vi "Instr_InitObject.vi"(8 "error in (no error)":errorcluster, 9 "Instrument Configuration":variant, 10 "Instrument address":refnum<visa-resource-name>, 11 "LXIPXISwitching in":refnum<class "LXIPXISwitching.lvclass">) -> (0 "error out":errorcluster, 3 "LXIPXISwitching out":refnum<class "LXIPXISwitching.lvclass">)   [LabVIEW 2019, in "LXIPXISwitching.lvclass"]
uses:
  LXIPXISwitching.lvclass
  InstrumentSetup.vi
  InstrControl.lvclass
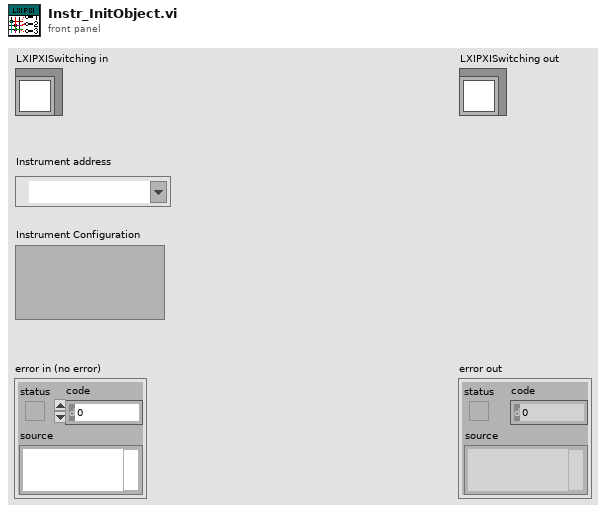
[diagram p1: front panel]
types:
  T1 = cluster{"MUX":string, "Matrix":string, "Breadboard":string, "LXIPXI Switching":refnum<class "LXIPXISwitching.lvclass">, "MUX PN":string, "Matrix  PN":string, "Breadboard PN":string, "MUX ID":string, "Matrix ID":string, "Breadboard ID":string, "LCR?":bool, "SMU?":bool}
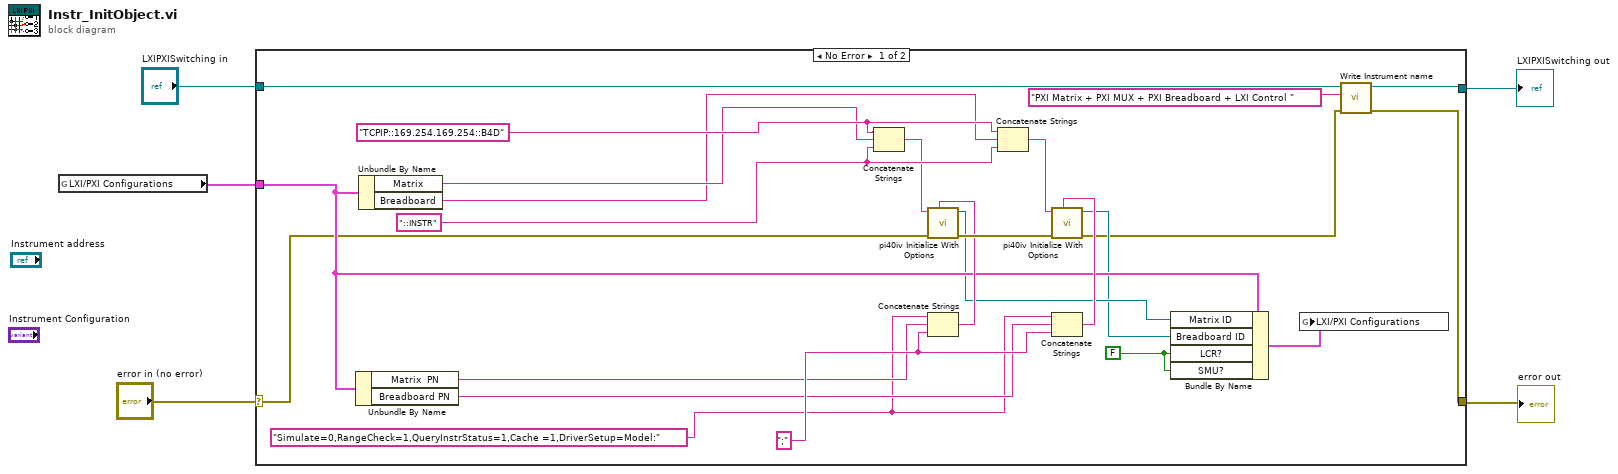
[diagram p0: block diagram]
diagram:
  n1 = global read "InstrumentSetup.vi" "LXI/PXI Configurations"() -> (w1:T1)
  n2 = case shown="No Error" "error in (no error)" {
    selector: "error in (no error)" -> [w6 w30]
    tunnel: [w9 w30] -> w4
    tunnel: [w12 w31] -> w2
    tunnel: "LXIPXISwitching in" -> [w11 w31]
    tunnel: w1 -> [w16 _]
    frame No Error {
      w7 = FALSE ("LCR?")
      w22 = "TCPIP::169.254.169.254::B4D"
      w19 = "::INSTR"
      w23 = "Simulate=0,RangeCheck=1,QueryInstrStatus=1,Cache =1,DriverSetup=Model:"
      w28 = ";" ("string")
      n3 = Unbundle By Name(w16) -> ("Matrix  PN"=w25:string, "Breadboard PN"=w24:string)
      n4 = Unbundle By Name(w16) -> ("Matrix"=w21:string, "Breadboard"=w20:string)
      n5 = Concatenate Strings(w22, w21, w19) -> (w18:string)
      n6 = Concatenate Strings(w23, w25, w28) -> (w27:string)
      n7 = call <instrlib>:"pi40iv Initialize With Options.vi"("option string"=w27, "error in (no error)"=w6, "resource name"=w18) -> ("error out"=w29:errorcluster, "instrument handle out"=w15:refnum<k15>)  [unwired: 7 in]
      n8 = Concatenate Strings(w22, w20, w19) -> (w17:string)
      n9 = Concatenate Strings(w23, w24, w28) -> (w26:string)
      n10 = call <instrlib>:"pi40iv Initialize With Options.vi"("option string"=w26, "error in (no error)"=w29, "resource name"=w17) -> ("error out"=w10:errorcluster, "instrument handle out"=w14:refnum<k15>)  [unwired: 7 in]
      n11 = Bundle By Name(cluster=w16, "Matrix ID"=w15, "Breadboard ID"=w14, "LCR?"=w7, "SMU?"=w7) -> (w13:T1)
      n12 = global write "InstrumentSetup.vi" "LXI/PXI Configurations"(w13) -> ()
      n13 = call-dynamic "Write Instrument name.vi"("error in (no error)"=w10, "Instrument name"="PXI Matrix + PXI MUX + PXI Breadboard + LXI Control ", "InstControl in"=w11) -> ("error out"=w9:errorcluster, "InstControl out"=w12:refnum<class "LXIPXISwitching.lvclass">)  [unwired: 7 in]
    }
    frame Error {
    }
  }
  "error out" <- w4
  "LXIPXISwitching out" <- w2
